vi "Main (test).vi"(11 "Array":dbl[](array[numeric])) -> (2 "X history":dbl[](array[numeric]), 3 "Y history":dbl[](array[numeric]))   [LabVIEW 2013]
panel:
  out "x Wall history":dbl[](array[numeric])
  out "y Wall history":dbl[](array[numeric])
  out "XY Graph":cluster{dbl[], dbl[]}[](graph)
  out "Heading history":dbl[](array[numeric])
  out "Encoder Right":dbl[](array[numeric])
  out "Encoder Left":dbl[](array[numeric])
  out "IR Front":dbl[](array[numeric])
  out "IR Right":dbl[](array[numeric])
  out "bot array":dbl[](array[numeric])
  in  "?":bool
  out "XBee string":string
  # "IR Right\n\nIR Front\n\nEncoder left\n\nEncoder righ"
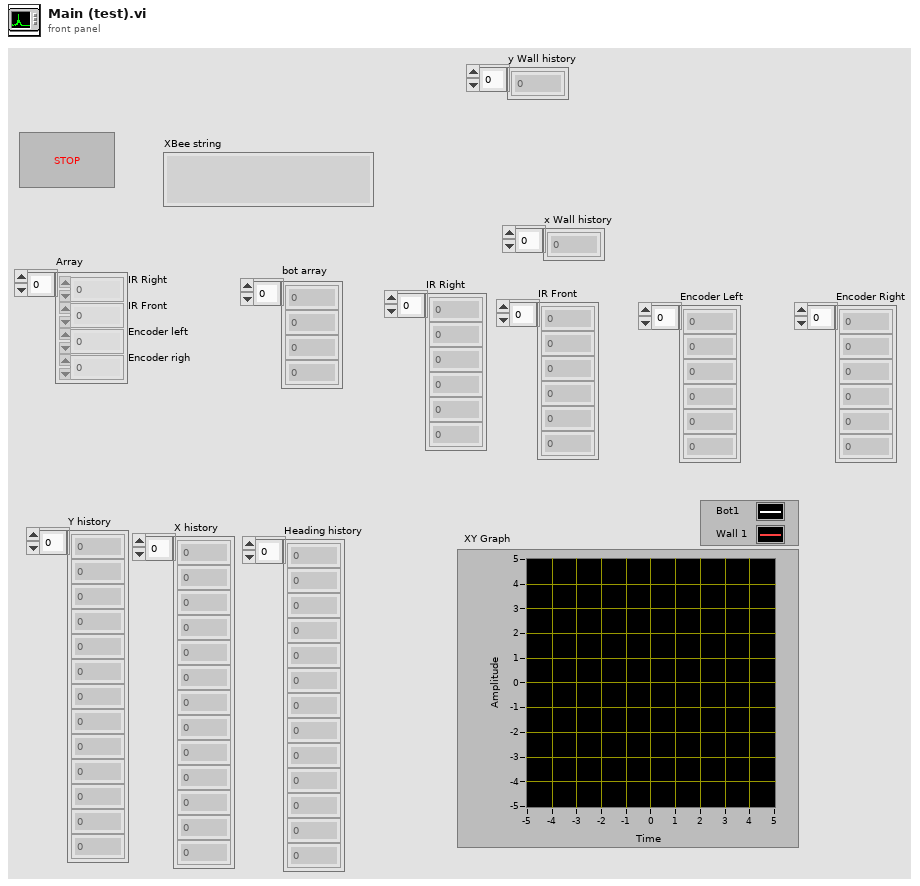
[diagram p1: front panel]
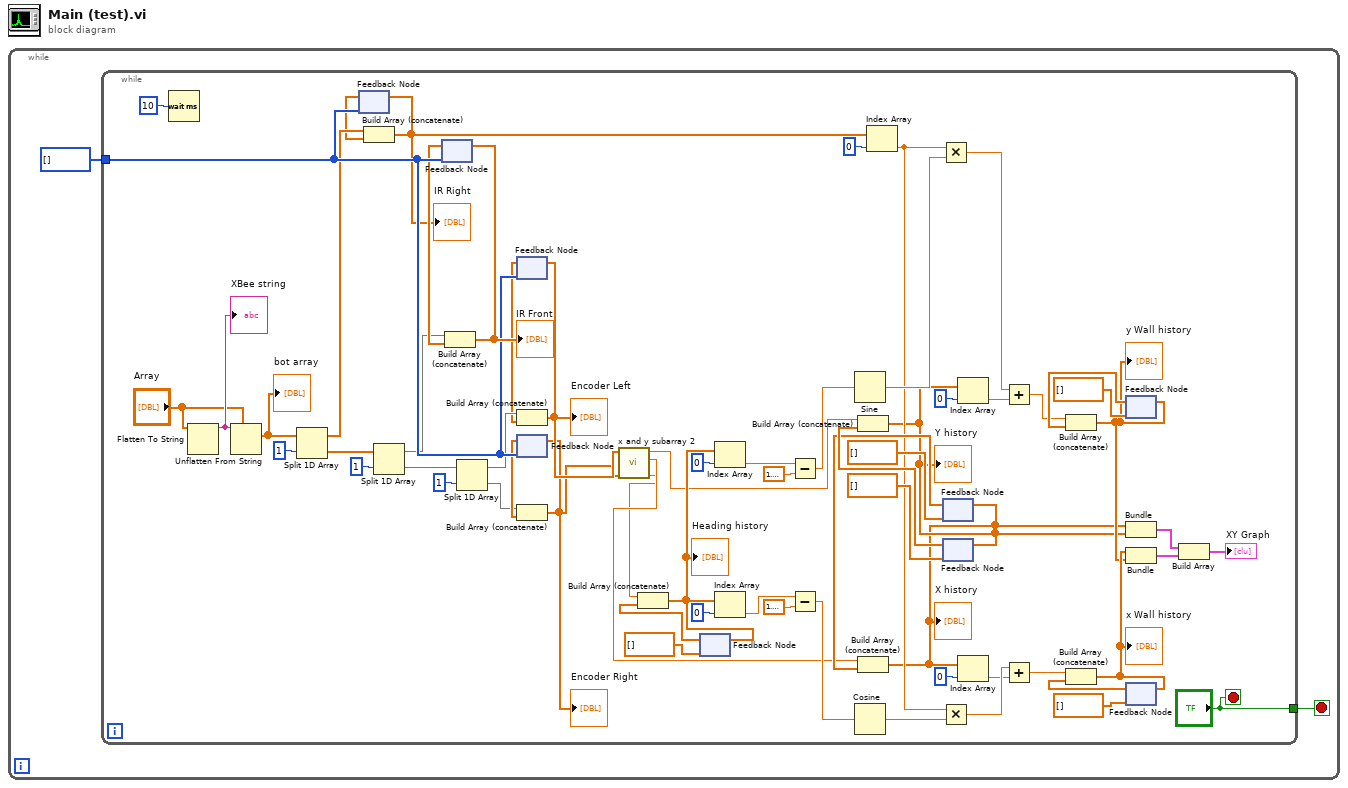
[diagram p0: block diagram]
diagram:
  n1 = while {
    stop <- w2 stop-if-true
    n2 = while {
      tunnel: ["?"] -> w2
      tunnel: i32[] [] -> [w55]
      stop <- "?" stop-if-true
      n3 = Wait (ms)(milliseconds to wait=u32 10) -> ()  [unwired: 1 out]
      n4 = Flatten To String(anything="Array") -> (data string=w66:string)  [unwired: 3 in, 2 out]
      "XBee string" <- w66
      n5 = Unflatten From String(type="Array", binary string=w66) -> (value=w64:dbl[])  [unwired: 3 in, 2 out]
      "bot array" <- w64
      n6 = Split 1D Array(array=w64, index=1) -> (first subarray=w48:dbl[], second subarray=w59:dbl[])
      n7 = feedback #1(w55) -> (w47:dbl[])
      n8 = Build Array (concatenate)(w48, w47) -> (w34:dbl[])
      "IR Right" <- w34
      n9 = feedback-in #1(w34) -> ()
      n10 = Split 1D Array(array=w59, index=1) -> (first subarray=w45:dbl[], second subarray=w60:dbl[])
      n11 = feedback #2(w55) -> (w46:dbl[])
      n12 = Build Array (concatenate)(w45, w46) -> (w56:dbl[])
      "IR Front" <- w56
      n13 = feedback-in #2(w56) -> ()
      n14 = Split 1D Array(array=w60, index=1) -> (first subarray=w44:dbl[], second subarray=w41:dbl[])
      n15 = feedback #3(w55) -> (w43:dbl[])
      n16 = Build Array (concatenate)(w44, w43) -> (w7:dbl[])
      "Encoder Left" <- w7
      n17 = feedback-in #3(w7) -> ()
      n18 = feedback #4(w55) -> (w42:dbl[])
      n19 = Build Array (concatenate)(w41, w42) -> (w6:dbl[])
      "Encoder Right" <- w6
      n20 = feedback-in #4(w6) -> ()
      n21 = call "x and y subarray 2.vi"("Encoder  Right"=w6, "Encoder Left"=w7) -> ("Heading"=w3:dbl, "x"=w5:dbl, "y"=w4:dbl)  [unwired: 7 in]
      n22 = feedback #5(dbl[] []) -> (w50:dbl[])
      n23 = Build Array (concatenate)(w3, w50) -> (w24:dbl[])
      "Heading history" <- w24
      n24 = feedback-in #5(w24) -> ()
      n25 = Index Array(array=w24, index=0) -> (element=w37:dbl)
      n26 = Index Array(array=w24, index=0) -> (element=w28:dbl)
      n27 = Subtract(x=w37, y=1.5707963267948966) -> (x-y=w36:dbl)
      n28 = Subtract(x=w28, y=1.5707963267948966) -> (x-y=w29:dbl)
      n29 = Sine(x=w36) -> (sin(x)=w40:dbl)
      n30 = Cosine(x=w29) -> (cos(x)=w26:dbl)
      n31 = Index Array(array=w34, index=0) -> (element=w18:dbl)
      n32 = Multiply(x=w18, y=w40) -> (x*y=w20:dbl)
      n33 = Multiply(x=w18, y=w26) -> (x*y=w14:dbl)
      n34 = feedback #6(dbl[] []) -> (w51:dbl[])
      n35 = Build Array (concatenate)(w5, w51) -> (w8:dbl[])
      "X history" <- w8
      n36 = feedback-in #6(w8) -> ()
      n37 = feedback #7(dbl[] []) -> (w54:dbl[])
      n38 = Build Array (concatenate)(w4, w54) -> (w9:dbl[])
      "Y history" <- w9
      n39 = feedback-in #7(w9) -> ()
      n40 = Index Array(array=w9, index=0) -> (element=w16:dbl)
      n41 = Index Array(array=w8, index=0) -> (element=w13:dbl)
      n42 = Add(x=w20, y=w16) -> (x+y=w19:dbl)
      n43 = Add(x=w14, y=w13) -> (x+y=w12:dbl)
      n44 = feedback #8(dbl[] []) -> (w33:dbl[])
      n45 = Build Array (concatenate)(w19, w33) -> (w10:dbl[])
      "y Wall history" <- w10
      n46 = feedback-in #8(w10) -> ()
      n47 = Bundle(w8, w9) -> (w23:cluster{dbl[], dbl[]})  [unwired: 1 in]
      n48 = feedback #9(dbl[] []) -> (w30:dbl[])
      n49 = Build Array (concatenate)(w12, w30) -> (w11:dbl[])
      "x Wall history" <- w11
      n50 = Bundle(w11, w10) -> (w22:cluster{dbl[], dbl[]})  [unwired: 1 in]
      n51 = feedback-in #9(w11) -> ()
      n52 = Build Array(w23, w22) -> (→"XY Graph":cluster{dbl[], dbl[]}[])
    }
  }
